vi "read_all_waveform_length.vi"(1 "N":i32, 2 "path":string) -> (0 "length":i32[](array[numeric]))   [LabVIEW 2022 SP3]
uses:
  <vilib>/Waveform/WDTFileIO.llb/Read Waveform from File.vi
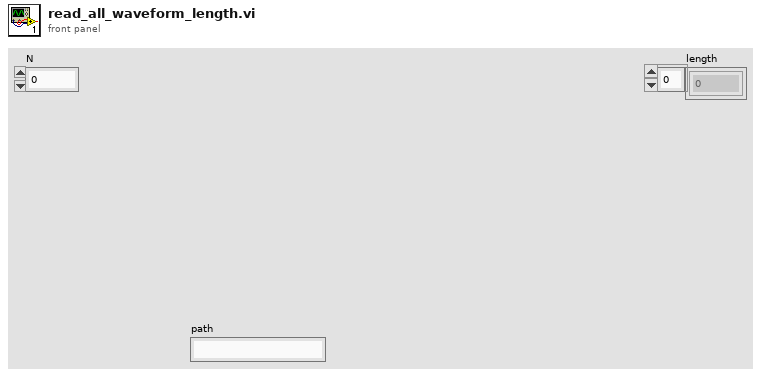
[diagram p1: front panel]
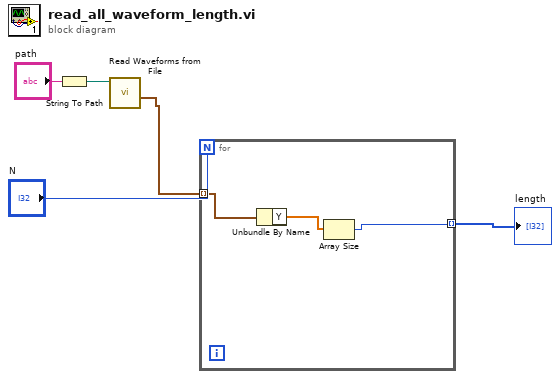
[diagram p0: block diagram]
diagram:
  n1 = String To Path(string="path") -> (path=w5:path)
  n2 = call-poly <vilib>:"Read Waveforms from File.vi"("file path (dialog if empty)"=w5) -> ("all waveforms in record"=w3:waveform(dbl)[])  [unwired: 5 in, 3 out]
  n3 = for {
    N: "N" -> [_]
    tunnel: w3 -> [w8] mode=indexing
    tunnel: [w6] -> w2 mode=indexing
    n4 = Unbundle By Name(w8) -> ("Y"=w7:dbl[])
    n5 = Array Size(array=w7) -> (size(s)=w6:i32)
  }
  "length" <- w2
